vi "timekeeper low pass filter.vi"(4 "Initialize":bool, 8 "offset":fxp<+/-,24,24>) -> (3 "filtered offset":fxp<+/-,24,24>)   [LabVIEW 2011, in "EPS_Timekeeper.lvlib"]
uses:
  <vilib>/addons/Electrical Power/Example Support/PMU/Time Keeper/EPS_Timekeeper.lvlib
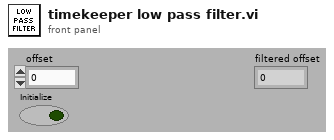
[diagram p1: front panel]
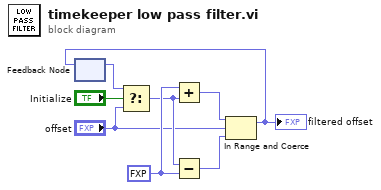
[diagram p0: block diagram]
diagram:
  w8 = fxp<+/-,18,18> 10000.0 ("x")
  n1 = feedback #1() -> (w7:fxp<+/-,24,24>)  [unwired: 1 in]
  n2 = Select(t=w7, s="Initialize", f="offset") -> (s? t:f=w3:fxp<+/-,24,24>)
  n3 = Add(x=w8, y=w3) -> (x+y=w6:fxp<+/-,18,18>)
  n4 = Subtract(x=w3, y=w8) -> (x-y=w5:fxp<+/-,18,18>)
  n5 = In Range and Coerce(upper limit=w6, x="offset", lower limit=w5) -> (coerced(x)=w4:fxp<+/-,24,24>)  [unwired: 1 out]
  "filtered offset" <- w4
  n6 = feedback-in #1(w4) -> ()
